vi "Start Sync.vi"(8 "error in (no error)":errorcluster, 11 "gRPC Server in":refnum<class "helloWServer.lvclass">) -> (0 "error out":errorcluster, 3 "gRPC Server out":refnum<class "helloWServer.lvclass">)   [LabVIEW 2020, in "helloWServer.lvlib" / "helloWServer.lvclass"]
uses:
  helloWServer.lvclass
  helloWServer.lvclass/helloWServer.ctl
  RPC Messages/helloworld_HelloReply/helloworld_HelloReply_Data.ctl
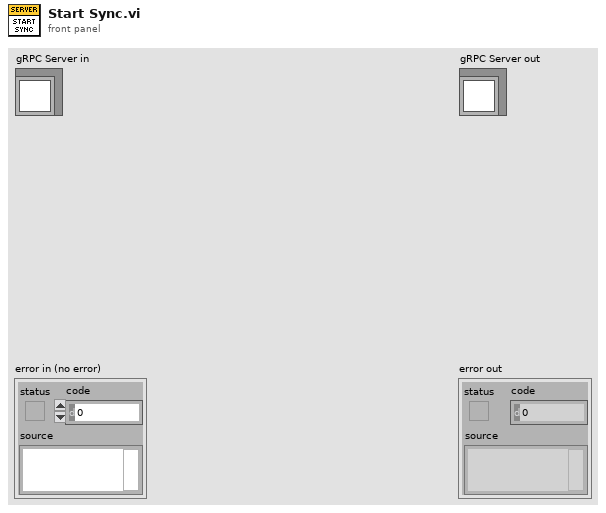
[diagram p1: front panel]
types:
  T1 = typedef "helloWServer.lvlib/helloWServer.lvclass/helloworld_HelloReply_Data.ctl" = cluster{"message":string}
  T2 = typedef "helloWServer.lvlib/helloWServer.lvclass/Server gRPC UEs.ctl" = cluster{"helloworld_Greeter_SayHello gRPC UE":refnum<user-event>}
  T3 = typedef "helloWServer.lvlib/gprc-lvsupport.lvlib/grpcId.ctl" = u64
  T4 = typedef "helloWServer.lvlib/helloWServer.lvclass/helloworld_HelloRequest_Data.ctl" = cluster{"name":string}
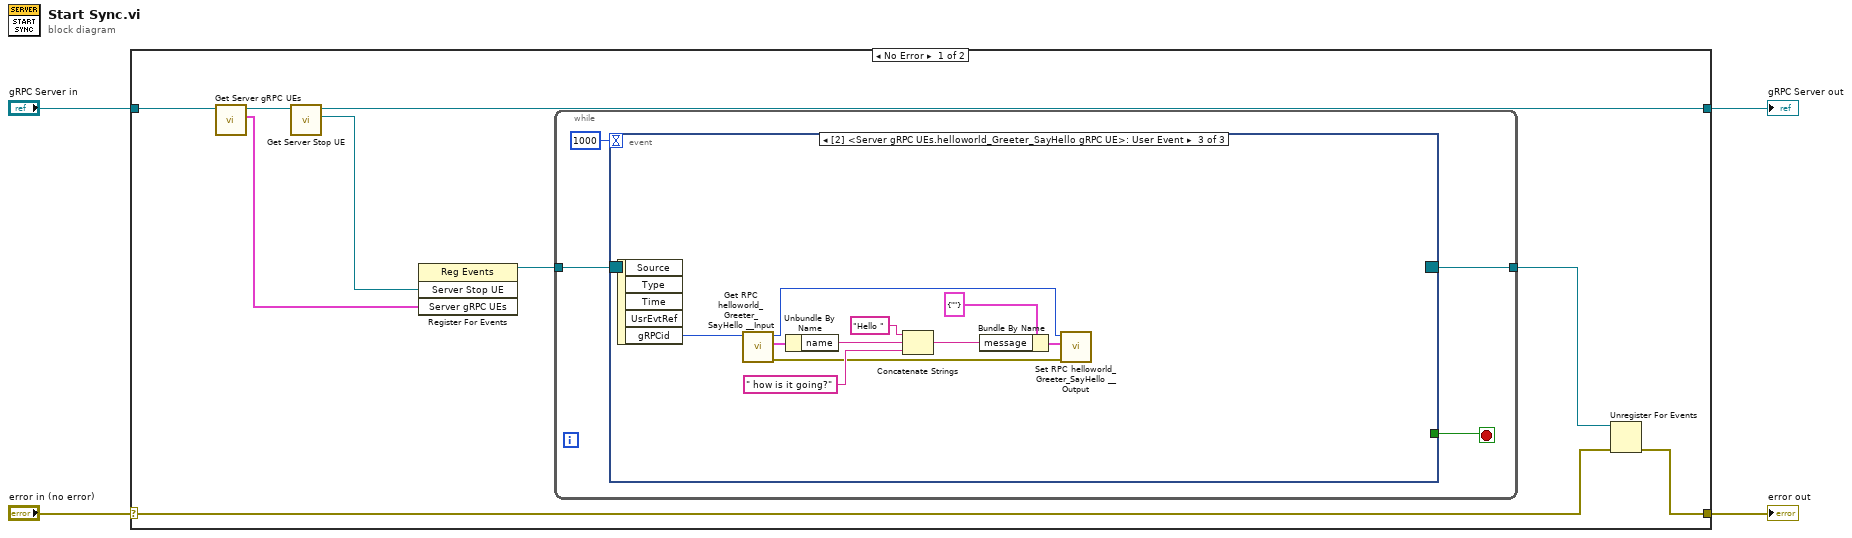
[diagram p0: block diagram]
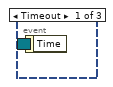
[diagram p2: hidden frame]
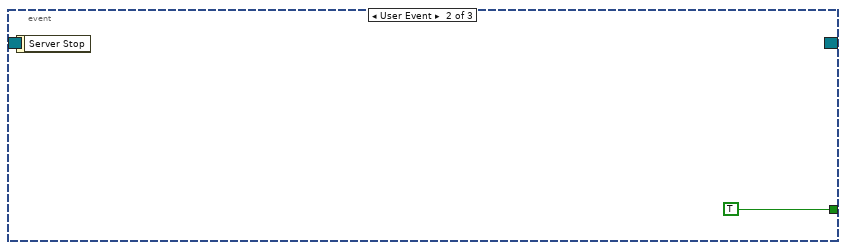
[diagram p3: hidden frame]
diagram:
  n1 = case shown="No Error" "error in (no error)" {
    selector: "error in (no error)" -> [w6 w30]
    tunnel: [w5 w30] -> w3
    tunnel: [w9 w29] -> w1
    tunnel: "gRPC Server in" -> [w13 w29]
    frame No Error {
      n2 = call "Get Server gRPC UEs.vi"("OOP Server in"=w13) -> ("Server gRPC UEs"=w10:T2, "OOP Server out"=w12:refnum<class "helloWServer.lvclass">)  [unwired: 9 in]
      n3 = call "Get Server Stop UE.vi"("OOP Server in"=w12) -> ("Server Stop UE"=w11:refnum<user-event>, "OOP Server out"=w9:refnum<class "helloWServer.lvclass">)  [unwired: 9 in]
      n4 = register-events(w11, w10) -> (reference out=w8:refnum<event-registration>)  [unwired: 2 in, 1 out]
      n5 = while {
        tunnel: w8 -> [w17]
        tunnel: [w15] -> w7
        stop <- w16 stop-if-true
        n6 = event "RPC Methods Event Structure" shown="[2] <Server gRPC UEs.helloworld_Greeter_SayHello gRPC UE>: User Event" {
          selector: w17 -> [_ _ _]
          dyn-events: [_ _ _] -> w15
          timeout: 1000 -> [_ _ _]
          tunnel: [_ TRUE _] -> w16
          event Timeout {
            n7 = event-data() -> ()  [unwired: 1 in, 1 out]
          }
          event User Event {
            n8 = event-data() -> ()  [unwired: 1 in, 1 out]
          }
          event User Event {
            n9 = event-data() -> ("gRPCid"=w28:T3)  [unwired: 1 in, 4 out]
            n10 = call "Get RPC helloworld_Greeter_SayHello __Input.vi"("gRPCid in"=w28) -> ("error out"=w19:errorcluster, "Message Data"=w27:T4, "gRPCid out"=w26:T3)  [unwired: 8 in]
            n11 = Unbundle By Name(w27) -> ("name"=w24:string)
            n12 = Concatenate Strings("Hello " ("string"), w24, " how is it going?" ("string")) -> (w21:string)
            n13 = Bundle By Name(cluster=T1 {"message"=""} ("Message Data"), "message"=w21) -> (w20:T1)
            n14 = call "Set RPC helloworld_Greeter_SayHello __Output.vi"("error in (no error)"=w19, "Message Data"=w20, "gRPCid in"=w26) -> ()  [unwired: 8 in, 1 out]
          }
        }
      }
      n15 = Unregister For Events(event registration refnum=w7, error in=w6) -> (error out=w5:errorcluster)
    }
    frame Error {
    }
  }
  "error out" <- w3
  "gRPC Server out" <- w1
